vi "Full Quit if Compiled.vi"(2 "stop/quit? (T)":bool) -> ()   [LabVIEW 2020, in "varilib.lvlib"]
doc: "If <b>not</b> in Run Time System: Stops the VI in which it executes, just as if you clicked the Abort Execution button on the toolbar. (Does not close all VIs, does not close LabVIEW).\nIf <b>in</b> Run Time System (compiled executable): Stops all executing VIs and ends the current instance of LabVIEW. (Close all VIs, stops the exe program)."
uses:
  varilib.lvlib
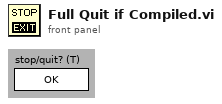
[diagram p1: front panel]
types:
  T1 = enum32{"invalid app kind", "Development System", "Run Time System", "Student Edition", "Embedded LabVIEW", "Evaluation", "Custom"}
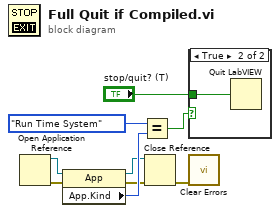
[diagram p0: block diagram]
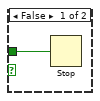
[diagram p2: hidden frame]
diagram:
  n1 = Open Application Reference() -> (0:w6:errorcluster, 3:w9:refnum<vi>)  [unwired: 4 in]
  n2 = property class="App"(reference=w9, error in=w6) -> (reference out=w4:refnum<vi>, error out=w5:errorcluster, "App.Kind"=w7:T1)
  n3 = Equal?(x=T1."Run Time System" ("Application:Kind"), y=w7) -> (x = y?=w2:bool)
  n4 = Close Reference(reference=w4, error in (no error)=w5) -> (error out=w3:errorcluster)
  n5 = case shown="True" w2 {
    tunnel: "stop/quit? (T)" -> [w10 w11]
    frame False {
      n6 = Stop(stop? (T)=w10) -> ()
    }
    frame True {
      n7 = Quit LabVIEW(quit? (T)=w11) -> ()
    }
  }
  n8 = call <vilib>:"Clear Errors.vi"("error in (no error)"=w3) -> ()  [unwired: 5 in, 2 out]
